vi "Quaternion to Euler.vi"(0 "Rotation Order":T2=enum."ZXY, 312", 1 "Quaternion":T3, 2 "Reference Frame":T1(ring)) -> (3 "R1":dbl, 4 "R2":dbl, 5 "R3":dbl, 6 "Singularity":bool)   [LabVIEW 2017]
uses:
  <vilib>/robotics/Kinematics/Quaternion.ctl
  <userlib>/836-Library/Sensor/IMU/Rot Order.ctl
  <vilib>/Analysis/baseanly.llb/Real Dot Product.vi
  <vilib>/Analysis/_algsub.llb/Vector Norm.vi
  <vilib>/Analysis/_algsub.llb/Real Vector Norm.vi
  <vilib>/robotics/Kinematics/Inverse Quaternion.vi
  <vilib>/robotics/Kinematics/Conjugate Quaternion.vi
  <vilib>/robotics/Kinematics/Multiply Quaternions.vi
  <vilib>/robotics/Kinematics/NI_Kinematics.lvlib
  <vilib>/Analysis/NI_AALBase.lvlib
  <vilib>/Analysis/NI_AALPro.lvlib
panel:
  out "Circular Order":bool
  out "Tait-Bryan":bool
  out "Proper Euler":bool
  # "Euler Angles"
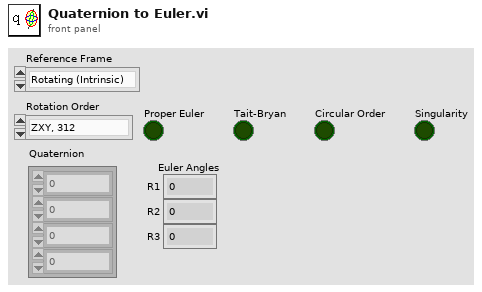
[diagram p1: front panel]
types:
  T1 = enum16{"Rotating (Intrinsic)", "Fixed (Extrinsic)"}
  T2 = typedef "Rot Order.ctl" = enum16{"ZXZ, 313", "XYX, 121", "YZY, 232", "ZYZ, 323", "XZX, 131", "YXY, 212", "XYZ, 123", "YZX, 231", "ZXY, 312", "XZY, 132", "ZYX, 321 NASA Standard Airplane", "YXZ, 213"}
  T3 = typedef "NI_Kinematics.lvlib/Quaternion.ctl" = dbl[]
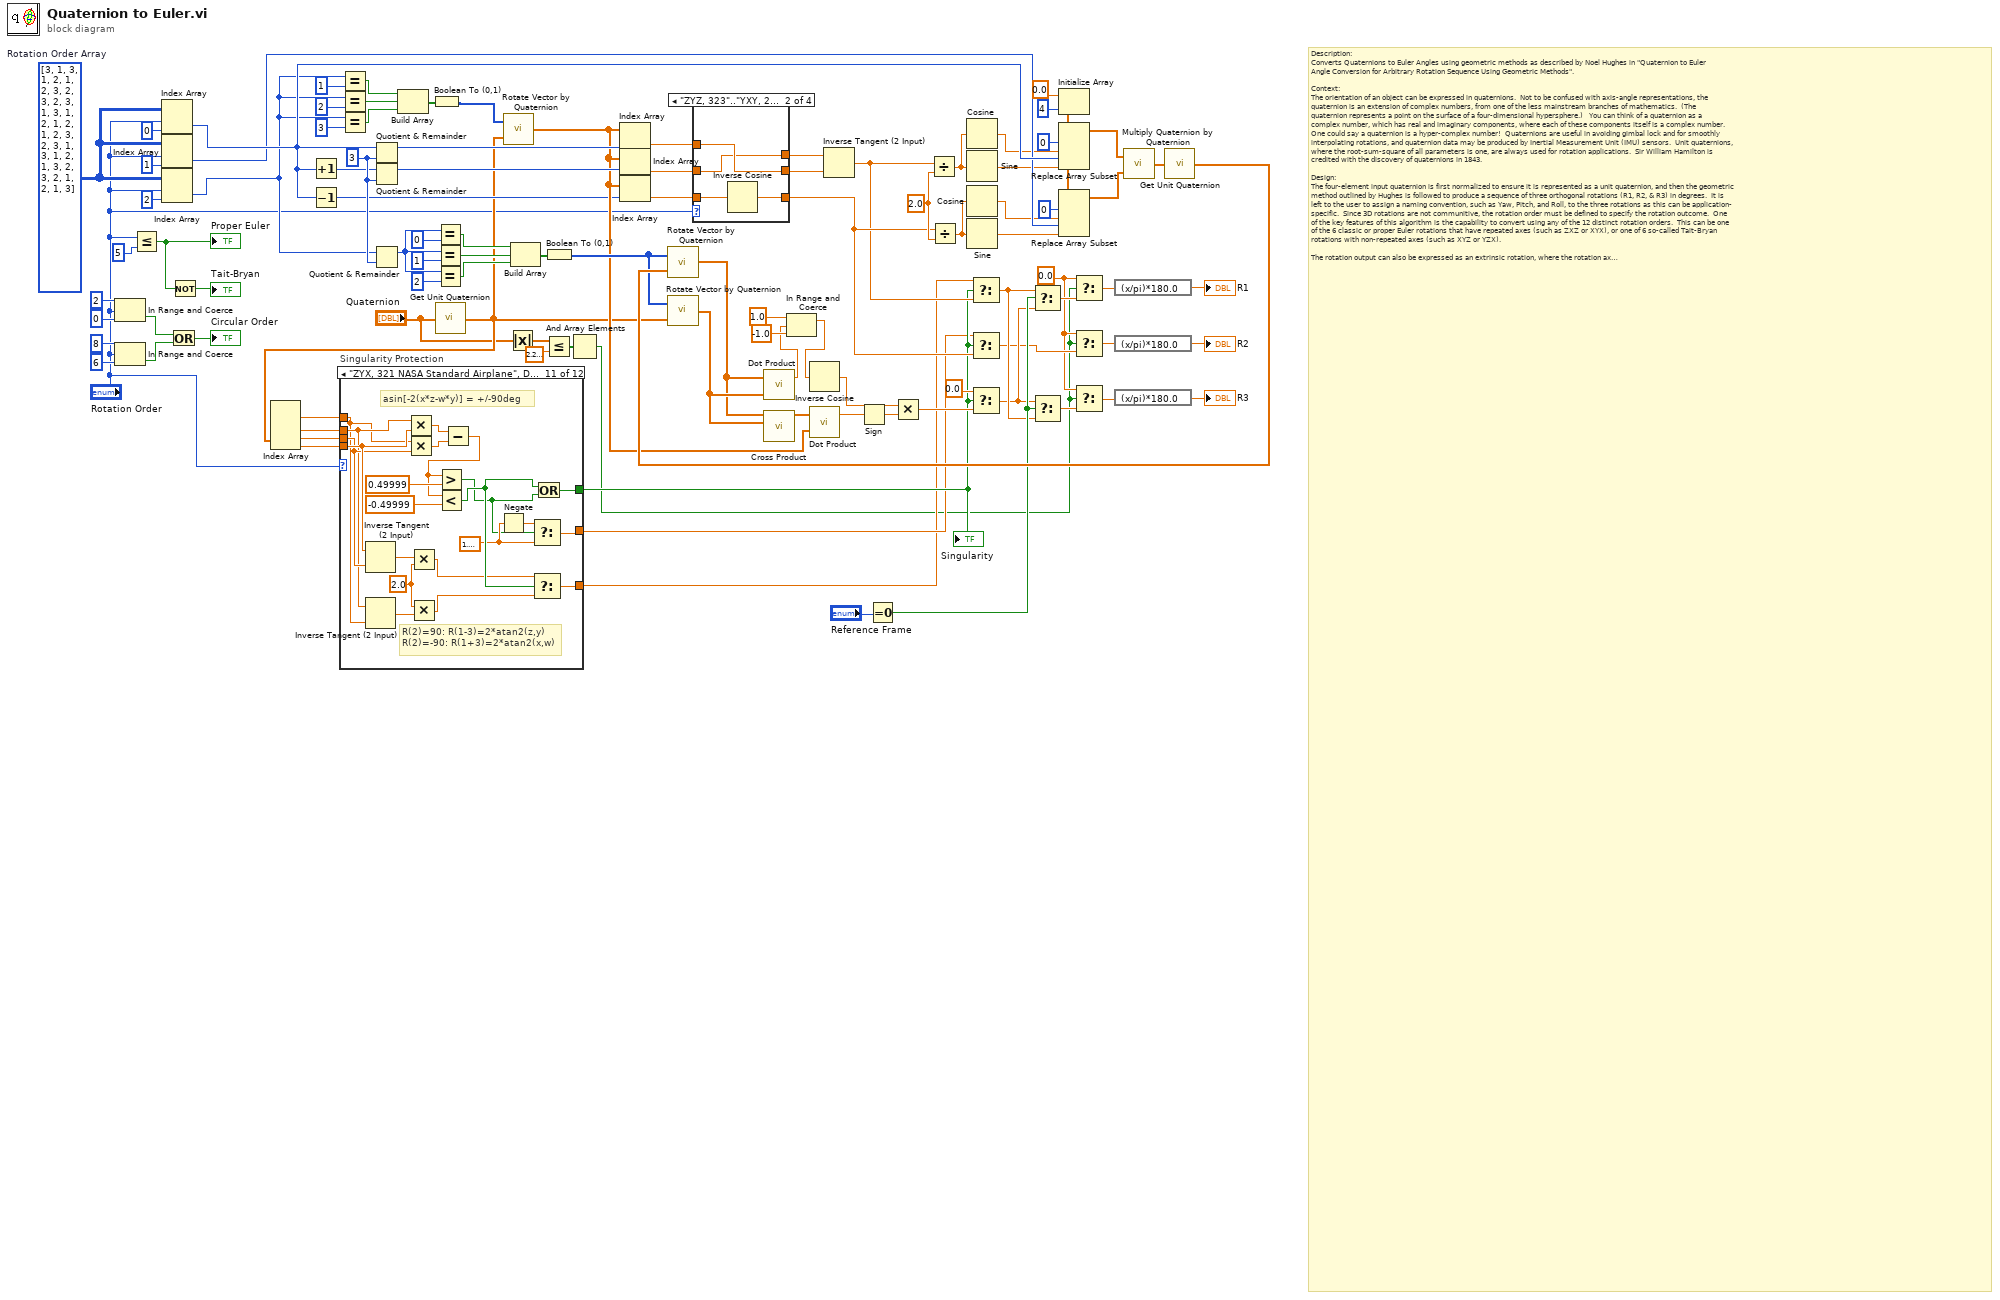
[diagram p0: block diagram]
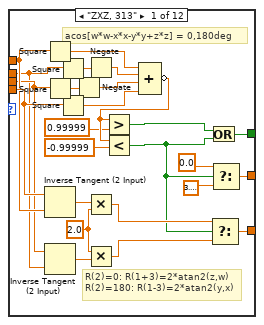
[diagram p2: hidden frame]
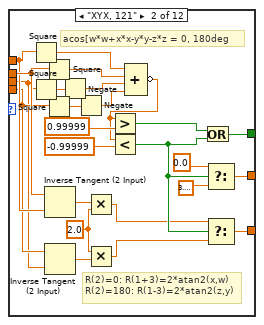
[diagram p3: hidden frame]
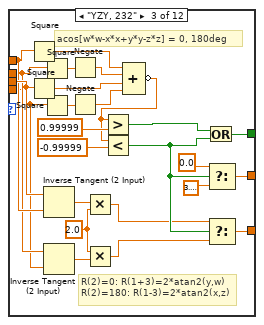
[diagram p4: hidden frame]
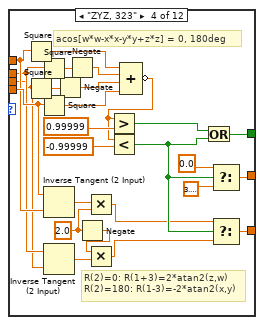
[diagram p5: hidden frame]
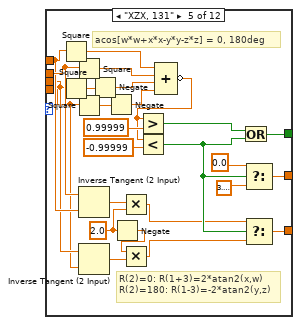
[diagram p6: hidden frame]
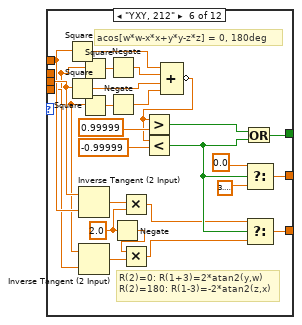
[diagram p7: hidden frame]
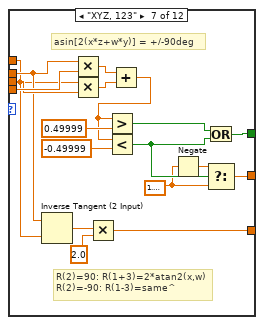
[diagram p8: hidden frame]
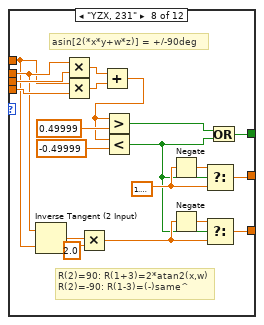
[diagram p9: hidden frame]
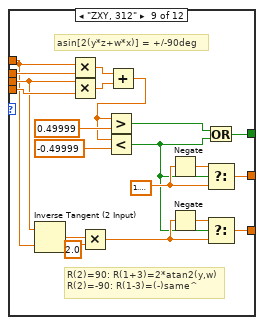
[diagram p10: hidden frame]
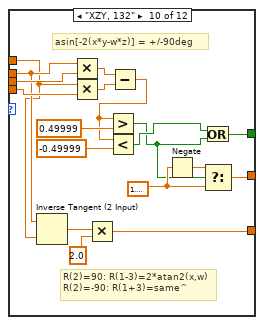
[diagram p11: hidden frame]
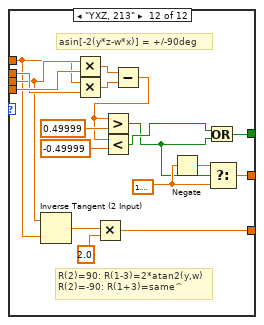
[diagram p12: hidden frame]
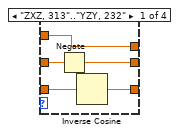
[diagram p13: hidden frame]
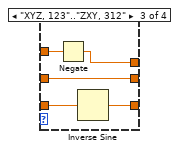
[diagram p14: hidden frame]
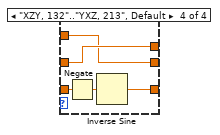
[diagram p15: hidden frame]
diagram:
  w7 = 0.0 ("t")
  w38 = 2.0 ("y")
  w75 = i16 3 ("y")
  w46 = i32[][] [[3, 1, 3], [1, 2, 1], [2, 3, 2], [3, 2, 3], [1, 3, 1], [2, 1, 2], [1, 2, 3], [2, 3, 1], [3, 1, 2], [1, 3, 2], [3, 2, 1], [2, 1, 3]]  # Rotation Order Array
  # "Description:\nConverts Quaternions to Euler Angles using geometric methods as described by Noel Hughes in \"Quaternion to Euler\nAngle Conversion for Arbitrary Rotation Sequence Using Geometric Methods\".\n\nContext:\nThe orientation of an object can be expressed in quaternions.  Not to be confused with axis-angle representations, the\nquaternion is an extension of complex numbers, from one of the less mainstream branches of mathematics.  (The\nquaternion represents a point on the surface of a four-dimensional hypersphere.)   You can think of a quaternion as a\ncomplex number, which has real and imaginary components, where each of these components itself is a complex number.\nOne could say a quaternion is a hyper-complex number!  Quaternions are useful in avoiding gimbal lock and for smoothly\ninterpolating rotations, and quaternion data may be produced by Inertial Measurement Unit (IMU) sensors.  Unit quaternions,\nwhere the root-sum-square of all parameters is one, are always used for rotation applications.  Sir William Hamilton is\ncredited with the discovery of quaternions in 1843. \n\nDesign:\nThe four-element input quaternion is first normalized to ensure it is represented as a unit quaternion, and then the geometric\nmethod outlined by Hughes is followed to produce a sequence of three orthogonal rotations (R1, R2, & R3) in degrees.  It is\nleft to the user to assign a naming convention, such as Yaw, Pitch, and Roll, to the three rotations as this can be application-\nspecific.  Since 3D rotations are not communitive, the rotation order must be defined to specify the rotation outcome.  One\nof the key features of this algorithm is the capability to convert using any of the 12 distinct rotation orders.  This can be one\nof the 6 classic or proper Euler rotations that have repeated axes (such as ZXZ or XYX), or one of 6 so-called Tait-Bryan\nrotations with non-repeated axes (such as XYZ or YZX).\n\nThe rotation output can also be expressed as an extrinsic rotation, where the rotation axes are the fixed world coordinate system,\nor an intrinsic rotation, using a coordinate system rotating with the rotating body.  Intrinsic rotations result in a changing\nreference system, where actual rotation axes might be X-Y'-Z\", for example, and are useful when the perspective is from the\nrotating body (such as an aircraft or robot).\n\nResearch determined the most elegant approach to performing this mathematically complicated conversion is described by this\nreference for a geometric conversion method by Mr. Noel Hughes:\n\n    http://www.euclideanspace.com/maths/geometry/rotations/conversions/quaternionToEuler/quat_2_euler_paper_ver2-1.pdf\n\nAll wire labels displayed in this implementation correspond to variable designations in Mr. Hughes document to facilitate\ncomparison.  Note that a different quaternion element structure is adopted here, [q0, q1i, q2j, q3k] where q0 is the real element,\nrather than [q1i, q2j, q3k, q4] where q4 is the real element (this is just a notation convention, and does not affect anything when\naccounted for).  This notation is also commonly understood as w,xi,yj,zk where 'w' is the real term coefficient.  Also note that\nequation 29 of the reference has been corrected to remove an unnecessary negative sign, and the reference equation 51 vector\nsubscript should be \"nG\" for clarity.\n\nFunctional additions to the referenced conversion approach, to provide robust coding, include :\n     (1)  a range coercion following the dot-product calculation to correct round-off error to avoid arccosine function error.\n     (2)  input value checking and mitigation for all-zero element quaternion to prevent NaN reporting in R1, R2, & R3.\n     (3)  singularity protection, which monitors for the ambiguity created when the second rotation aligns the first and third \n            rotation axes (AKA Gimbal Lock).\n\nInputs:\nQUATERNION - Input quaternion for conversion to Euler Angles.\nROTATION ORDER - Order of axis rotation used for conversion.\nREFERENCE FRAME - Designation of perspective, world coordinate system/extrinsic/fixed reference frame, or \n                                      body coordinate system/intrinsic/rotating reference frame.\n\nOutputs:\nEULER ANGLES - Cluster containing computed first, second, and third rotations (R1, R2, & R3) as converted from input quaternion. \nSINGULARITY - Boolean indicating if singularity (gimbal lock) is detected.\nPROPER EULER - Boolean indicating if rotation order is of the Proper/Classic form, (diagnostic).\nTAIT-BRYAN - Boolean indicating if rotation order is of the Tait-Bryan form, (diagnostic).\nCIRCULAR ORDER - Boolean indicating if rotation axes are in circular order, i.e. 123, 231, or 312, (diagnostic).\n\n\nVI Properties:\nExecution Reentrancy is set to Non-Reentrant Execution\n\nImplementation Considerations:\nA mathematical ambiguity can occur when the second rotation aligns the axes of the first and third rotation, also known as gimbal\nlock.  When this occurs, a degree of freedom is lost and the first and third axis rotations are indistinguishable and each produce\nthe same effect.  This is not a defect of the conversion approach or coding, but a topological result of representing 3D rotations\nwith Euler Angles.  This implementation handles the ambiguity by associating all first/third axis rotation to R1, and setting R3 to\nzero (since their respective contributions are otherwise unresolvable).  This approach is arbitrary but evidently in keeping with\ngeneral convention.  The Singularity Protection Case Structure monitors for this condition as a function of each of the 12 distinct\nrotation orders.  The way to read the notes within each case, using rotation order \"ZYX\" as an example, is:\n\n      Singularity will occur when sin[-2(x*z-w*y)] is either +90 or -90 degrees (one is Pitched North and one South).  When this\n      occurs, rotation 2 will be either +/-90 degrees, and rotations 1 and 3 are indistinguishable.  However, if R2 is +90, then we \n      know that the difference R1-R3 will equal 2*atan2(z,y).  When R2 is -90, we know that the sum R1+R3 will equal 2*atan2(x,w).\n\nEach rotation order requires a different derivation for these formulas.  The R1/R3 combination is all arbitrarily assigned to R1,\nand R3 is set to zero.  These equations were derived by this author, separately from the reference document (any errors are mine).\n\nThe implication is that under the conditions of singularity, only the second rotation R2 can be explicitly trusted to align with reality.\nThe Singularity output Boolean is available to indicate when this condition occurs.\n\n\n----- The RoboBees FRC Team 836! -----  Even hyper-complex numbers can be tamed!! ... get hyper about a career in STEM!"
  n1 = In Range and Coerce(upper limit=2, x="Rotation Order", lower limit=0) -> (In Range?=w55:bool)  [unwired: 1 out]
  n2 = In Range and Coerce(upper limit=8, x="Rotation Order", lower limit=6) -> (In Range?=w56:bool)  [unwired: 1 out]
  n3 = Less Or Equal?(x="Rotation Order", y=5) -> (x <= y?=w50:bool)
  "Proper Euler" <- w50
  n4 = Index Array(array=w46, index (row)="Rotation Order", index (col)=0 ("disabled index (col)")) -> (element=w103:i32)
  n5 = Index Array(array=w46, index (row)="Rotation Order", index (col)=1 ("disabled index (col)")) -> (element=w95:i32)
  n6 = Index Array(array=w46, index (row)="Rotation Order", index (col)=2 ("disabled index (col)")) -> (element=w74:i32)
  n7 = Or(x=w55, y=w56) -> (x .or. y?=→"Circular Order":bool)
  n8 = Not(x=w50) -> (.not. x?=→"Tait-Bryan":bool)
  n9 = Increment(x=w103) -> (x+1=w70:i32)
  n10 = Decrement(x=w103) -> (x-1=w65:i32)
  n11 = Equal?(x=w74, y=1) -> (x = y?=w62:bool)
  n12 = Equal?(x=w74, y=2) -> (x = y?=w61:bool)
  n13 = Equal?(x=w74, y=3) -> (x = y?=w63:bool)
  n14 = Quotient & Remainder(x=w103, y=w75) -> (x-y*floor(x/y)=w71:i32)  [unwired: 1 out]
  n15 = Quotient & Remainder(x=w70, y=w75) -> (x-y*floor(x/y)=w72:i32)  [unwired: 1 out]
  n16 = Quotient & Remainder(x=w74, y=w75) -> (x-y*floor(x/y)=w83:i32)  [unwired: 1 out]
  n17 = Build Array(w62, w61, w63) -> (w64:bool[])
  n18 = Boolean To (0,1)(Boolean=w64) -> (0, 1=w73:i16[])
  n19 = Equal?(x=w83, y=0) -> (x = y?=w78:bool)
  n20 = Equal?(x=w83, y=1) -> (x = y?=w79:bool)
  n21 = Equal?(x=w83, y=2) -> (x = y?=w77:bool)
  n22 = call <vilib>:"Get Unit Quaternion.vi"("quaternion"="Quaternion") -> ("unit quaternion"=w33:T3)
  n23 = Index Array(array=w33) -> (element #1=w29:dbl, element #2=w28:dbl, element #3=w30:dbl, element #4=w31:dbl)  [unwired: 4 in]
  n24 = case "Singularity Protection" shown="\"ZYX, 321 NASA Standard Airplane\", Default" "Rotation Order" {
    tunnel: w29 -> [w114 w140 w164 w192 w215 w241 w264 w283 w303 w322 w341 w361]
    tunnel: w28 -> [w112 w141 w163 w191 w216 w239 w265 w284 w311 w323 w342 w368]
    tunnel: w30 -> [w113 w138 w165 w190 w214 w242 w271 w292 w304 w330 w343 w362]
    tunnel: w31 -> [w115 w139 w162 w193 w213 w240 w272 w291 w312 w329 w344 w369]
    tunnel: [w109 w131 w155 w181 w209 w234 w259 w276 w296 w316 w335 w355] -> w21
    tunnel: [w116 w137 w166 w189 w217 w243 w261 w285 w302 w319 w345 w358] -> w20
    tunnel: [w110 w136 w161 w186 w212 w237 w263 w281 w301 w321 w340 w360] -> w22
    frame "ZXZ, 313" {
      w118 = 2.0 ("y")
      # "acos[w*w-x*x-y*y+z*z] = 0,180deg"
      # "R(2)=0: R(1+3)=2*atan2(z,w)\nR(2)=180: R(1-3)=2*atan2(y,x)"
      n25 = Square(x=w114) -> (x^2=w125:dbl)
      n26 = Square(x=w113) -> (x^2=w124:dbl)
      n27 = Inverse Tangent (2 Input)(1:w114, 2:w115) -> (0:w119:dbl)
      n28 = Inverse Tangent (2 Input)(1:w112, 2:w113) -> (0:w117:dbl)
      n29 = Square(x=w112) -> (x^2=w123:dbl)
      n30 = Square(x=w115) -> (x^2=w128:dbl)
      n31 = Negate(x=w124) -> (-x=w127:dbl)
      n32 = Negate(x=w123) -> (-x=w126:dbl)
      n33 = Multiply(x=w119, y=w118) -> (x*y=w108:dbl)
      n34 = Multiply(x=w118, y=w117) -> (x*y=w107:dbl)
      n35 = Compound Arithmetic op=ADD(w125, w126, w127, w128) -> (invert w121:dbl)
      n36 = Greater?(x=w121, y=0.99999 ("upper limit")) -> (0:w111:bool)
      n37 = Less?(x=w121, y=-0.99999 ("lower limit")) -> (x < y?=w106:bool)
      n38 = Or(x=w111, y=w106) -> (x .or. y?=w110:bool)
      n39 = Select(t=w108, s=w106, f=w107) -> (s? t:f=w116:dbl)
      n40 = Select(t=0.0 ("f"), s=w106, f=3.141592653589793) -> (s? t:f=w109:dbl)
    }
    frame "XYX, 121" {
      w143 = 2.0 ("y")
      # "R(2)=0: R(1+3)=2*atan2(x,w)\nR(2)=180: R(1-3)=2*atan2(z,y)"
      # "acos[w*w+x*x-y*y-z*z = 0, 180deg"
      n41 = Square(x=w140) -> (x^2=w152:dbl)
      n42 = Square(x=w138) -> (x^2=w151:dbl)
      n43 = Square(x=w141) -> (x^2=w148:dbl)
      n44 = Square(x=w139) -> (x^2=w150:dbl)
      n45 = Inverse Tangent (2 Input)(1:w140, 2:w141) -> (0:w144:dbl)
      n46 = Inverse Tangent (2 Input)(1:w138, 2:w139) -> (0:w142:dbl)
      n47 = Negate(x=w151) -> (-x=w153:dbl)
      n48 = Negate(x=w150) -> (-x=w149:dbl)
      n49 = Multiply(x=w144, y=w143) -> (x*y=w130:dbl)
      n50 = Multiply(x=w143, y=w142) -> (x*y=w129:dbl)
      n51 = Compound Arithmetic op=ADD(w152, w148, w153, w149) -> (invert w145:dbl)
      n52 = Greater?(x=w145, y=0.99999 ("upper limit")) -> (0:w135:bool)
      n53 = Less?(x=w145, y=-0.99999 ("lower limit")) -> (x < y?=w133:bool)
      n54 = Or(x=w135, y=w133) -> (x .or. y?=w136:bool)
      n55 = Select(t=0.0 ("f"), s=w133, f=3.141592653589793) -> (s? t:f=w131:dbl)
      n56 = Select(t=w130, s=w133, f=w129) -> (s? t:f=w137:dbl)
    }
    frame "YZY, 232" {
      w168 = 2.0 ("y")
      # "R(2)=0: R(1+3)=2*atan2(y,w)\nR(2)=180: R(1-3)=2*atan2(x,z)"
      # "acos[w*w-x*x+y*y-z*z] = 0, 180deg"
      n57 = Square(x=w164) -> (x^2=w177:dbl)
      n58 = Square(x=w165) -> (x^2=w173:dbl)
      n59 = Square(x=w163) -> (x^2=w176:dbl)
      n60 = Square(x=w162) -> (x^2=w175:dbl)
      n61 = Inverse Tangent (2 Input)(1:w164, 2:w165) -> (0:w169:dbl)
      n62 = Inverse Tangent (2 Input)(1:w162, 2:w163) -> (0:w167:dbl)
      n63 = Negate(x=w176) -> (-x=w178:dbl)
      n64 = Negate(x=w175) -> (-x=w174:dbl)
      n65 = Multiply(x=w169, y=w168) -> (x*y=w157:dbl)
      n66 = Multiply(x=w168, y=w167) -> (x*y=w156:dbl)
      n67 = Compound Arithmetic op=ADD(w177, w178, w173, w174) -> (invert w170:dbl)
      n68 = Greater?(x=w170, y=0.99999 ("upper limit")) -> (0:w160:bool)
      n69 = Less?(x=w170, y=-0.99999 ("lower limit")) -> (x < y?=w158:bool)
      n70 = Or(x=w160, y=w158) -> (x .or. y?=w161:bool)
      n71 = Select(t=0.0 ("f"), s=w158, f=3.141592653589793) -> (s? t:f=w155:dbl)
      n72 = Select(t=w157, s=w158, f=w156) -> (s? t:f=w166:dbl)
    }
    frame "ZYZ, 323" {
      w188 = 2.0 ("y")
      # "R(2)=0: R(1+3)=2*atan2(z,w)\nR(2)=180: R(1-3)=-2*atan2(x,y)"
      # "acos[w*w-x*x-y*y+z*z] = 0, 180deg"
      n73 = Square(x=w192) -> (x^2=w201:dbl)
      n74 = Square(x=w190) -> (x^2=w200:dbl)
      n75 = Square(x=w191) -> (x^2=w199:dbl)
      n76 = Square(x=w193) -> (x^2=w204:dbl)
      n77 = Inverse Tangent (2 Input)(1:w192, 2:w193) -> (0:w195:dbl)
      n78 = Inverse Tangent (2 Input)(1:w190, 2:w191) -> (0:w194:dbl)
      n79 = Negate(x=w200) -> (-x=w203:dbl)
      n80 = Negate(x=w199) -> (-x=w202:dbl)
      n81 = Negate(x=w188) -> (-x=w187:dbl)
      n82 = Multiply(x=w195, y=w188) -> (x*y=w180:dbl)
      n83 = Multiply(x=w187, y=w194) -> (x*y=w179:dbl)
      n84 = Compound Arithmetic op=ADD(w201, w202, w203, w204) -> (invert w196:dbl)
      n85 = Greater?(x=w196, y=0.99999 ("upper limit")) -> (0:w185:bool)
      n86 = Less?(x=w196, y=-0.99999 ("lower limit")) -> (x < y?=w183:bool)
      n87 = Or(x=w185, y=w183) -> (x .or. y?=w186:bool)
      n88 = Select(t=0.0 ("f"), s=w183, f=3.141592653589793) -> (s? t:f=w181:dbl)
      n89 = Select(t=w180, s=w183, f=w179) -> (s? t:f=w189:dbl)
    }
    frame "XZX, 131" {
      w219 = 2.0 ("y")
      # "R(2)=0: R(1+3)=2*atan2(x,w)\nR(2)=180: R(1-3)=-2*atan2(y,z)"
      # "acos[w*w+x*x-y*y-z*z] = 0, 180deg"
      n90 = Square(x=w215) -> (x^2=w229:dbl)
      n91 = Square(x=w214) -> (x^2=w228:dbl)
      n92 = Square(x=w216) -> (x^2=w225:dbl)
      n93 = Square(x=w213) -> (x^2=w227:dbl)
      n94 = Inverse Tangent (2 Input)(1:w215, 2:w216) -> (0:w221:dbl)
      n95 = Inverse Tangent (2 Input)(1:w213, 2:w214) -> (0:w220:dbl)
      n96 = Negate(x=w228) -> (-x=w230:dbl)
      n97 = Negate(x=w227) -> (-x=w226:dbl)
      n98 = Negate(x=w219) -> (-x=w218:dbl)
      n99 = Multiply(x=w221, y=w219) -> (x*y=w206:dbl)
      n100 = Multiply(x=w218, y=w220) -> (x*y=w205:dbl)
      n101 = Compound Arithmetic op=ADD(w229, w225, w230, w226) -> (invert w222:dbl)
      n102 = Greater?(x=w222, y=0.99999 ("upper limit")) -> (0:w211:bool)
      n103 = Less?(x=w222, y=-0.99999 ("lower limit")) -> (x < y?=w208:bool)
      n104 = Or(x=w211, y=w208) -> (x .or. y?=w212:bool)
      n105 = Select(t=0.0 ("f"), s=w208, f=3.141592653589793) -> (s? t:f=w209:dbl)
      n106 = Select(t=w206, s=w208, f=w205) -> (s? t:f=w217:dbl)
    }
    frame "YXY, 212" {
      w245 = 2.0 ("y")
      # "R(2)=0: R(1+3)=2*atan2(y,w)\nR(2)=180: R(1-3)=-2*atan2(z,x)"
      # "acos[w*w-x*x+y*y-z*z] = 0, 180deg"
      n107 = Square(x=w241) -> (x^2=w255:dbl)
      n108 = Square(x=w242) -> (x^2=w251:dbl)
      n109 = Inverse Tangent (2 Input)(1:w241, 2:w242) -> (0:w247:dbl)
      n110 = Inverse Tangent (2 Input)(1:w239, 2:w240) -> (0:w246:dbl)
      n111 = Square(x=w239) -> (x^2=w254:dbl)
      n112 = Square(x=w240) -> (x^2=w253:dbl)
      n113 = Negate(x=w254) -> (-x=w256:dbl)
      n114 = Negate(x=w253) -> (-x=w252:dbl)
      n115 = Negate(x=w245) -> (-x=w244:dbl)
      n116 = Multiply(x=w247, y=w245) -> (x*y=w232:dbl)
      n117 = Multiply(x=w244, y=w246) -> (x*y=w231:dbl)
      n118 = Compound Arithmetic op=ADD(w255, w256, w251, w252) -> (invert w248:dbl)
      n119 = Greater?(x=w248, y=0.99999 ("upper limit")) -> (0:w238:bool)
      n120 = Less?(x=w248, y=-0.99999 ("lower limit")) -> (x < y?=w233:bool)
      n121 = Or(x=w238, y=w233) -> (x .or. y?=w237:bool)
      n122 = Select(t=0.0 ("f"), s=w233, f=3.141592653589793) -> (s? t:f=w234:dbl)
      n123 = Select(t=w232, s=w233, f=w231) -> (s? t:f=w243:dbl)
    }
    frame "XYZ, 123" {
      w257 = 1.5707963267948966
      # "R(2)=90: R(1+3)=2*atan2(x,w)\nR(2)=-90: R(1-3)=same^"
      # "asin[2(x*z+w*y)] = +/-90deg"
      n124 = Inverse Tangent (2 Input)(1:w264, 2:w265) -> (0:w267:dbl)
      n125 = Multiply(x=w265, y=w272) -> (x*y=w274:dbl)
      n126 = Multiply(x=w264, y=w271) -> (x*y=w273:dbl)
      n127 = Multiply(x=w267, y=2.0) -> (x*y=w261:dbl)
      n128 = Add(x=w274, y=w273) -> (x+y=w268:dbl)
      n129 = Greater?(x=w268, y=0.49999 ("upper limit")) -> (0:w262:bool)
      n130 = Less?(x=w268, y=-0.49999 ("lower limit")) -> (x < y?=w260:bool)
      n131 = Negate(x=w257) -> (-x=w258:dbl)
      n132 = Or(x=w262, y=w260) -> (x .or. y?=w263:bool)
      n133 = Select(t=w258, s=w260, f=w257) -> (s? t:f=w259:dbl)
    }
    frame "YZX, 231" {
      w277 = 1.5707963267948966
      # "R(2)=90: R(1+3)=2*atan2(x,w)\nR(2)=-90: R(1-3)=(-)same^"
      # "asin[2(*x*y+w*z)] = +/-90deg"
      n134 = Inverse Tangent (2 Input)(1:w283, 2:w284) -> (0:w287:dbl)
      n135 = Multiply(x=w284, y=w292) -> (x*y=w293:dbl)
      n136 = Multiply(x=w283, y=w291) -> (x*y=w294:dbl)
      n137 = Multiply(x=w287, y=2.0) -> (x*y=w279:dbl)
      n138 = Add(x=w293, y=w294) -> (x+y=w288:dbl)
      n139 = Greater?(x=w288, y=0.49999 ("upper limit")) -> (0:w280:bool)
      n140 = Less?(x=w288, y=-0.49999 ("lower limit")) -> (x < y?=w275:bool)
      n141 = Negate(x=w277) -> (-x=w278:dbl)
      n142 = Negate(x=w279) -> (-x=w282:dbl)
      n143 = Select(t=w278, s=w275, f=w277) -> (s? t:f=w276:dbl)
      n144 = Select(t=w282, s=w275, f=w279) -> (s? t:f=w285:dbl)
      n145 = Or(x=w280, y=w275) -> (x .or. y?=w281:bool)
    }
    frame "ZXY, 312" {
      w297 = 1.5707963267948966
      # "R(2)=90: R(1+3)=2*atan2(y,w)\nR(2)=-90: R(1-3)=(-)same^"
      # "asin[2(y*z+w*x)] = +/-90deg"
      n146 = Inverse Tangent (2 Input)(1:w303, 2:w304) -> (0:w307:dbl)
      n147 = Multiply(x=w303, y=w311) -> (x*y=w314:dbl)
      n148 = Multiply(x=w304, y=w312) -> (x*y=w313:dbl)
      n149 = Multiply(x=w307, y=2.0) -> (x*y=w299:dbl)
      n150 = Add(x=w314, y=w313) -> (x+y=w308:dbl)
      n151 = Greater?(x=w308, y=0.49999 ("upper limit")) -> (0:w300:bool)
      n152 = Less?(x=w308, y=-0.49999 ("lower limit")) -> (x < y?=w295:bool)
      n153 = Negate(x=w297) -> (-x=w298:dbl)
      n154 = Negate(x=w299) -> (-x=w305:dbl)
      n155 = Or(x=w300, y=w295) -> (x .or. y?=w301:bool)
      n156 = Select(t=w298, s=w295, f=w297) -> (s? t:f=w296:dbl)
      n157 = Select(t=w305, s=w295, f=w299) -> (s? t:f=w302:dbl)
    }
    frame "XZY, 132" {
      w317 = 1.5707963267948966
      # "R(2)=90: R(1-3)=2*atan2(x,w)\nR(2)=-90: R(1+3)=same^"
      # "asin[-2(x*y-w*z)] = +/-90deg"
      n158 = Inverse Tangent (2 Input)(1:w322, 2:w323) -> (0:w325:dbl)
      n159 = Multiply(x=w323, y=w330) -> (x*y=w332:dbl)
      n160 = Multiply(x=w322, y=w329) -> (x*y=w331:dbl)
      n161 = Multiply(x=w325, y=2.0) -> (x*y=w319:dbl)
      n162 = Subtract(x=w332, y=w331) -> (x-y=w326:dbl)
      n163 = Greater?(x=w326, y=0.49999 ("upper limit")) -> (0:w315:bool)
      n164 = Less?(x=w326, y=-0.49999 ("lower limit")) -> (x < y?=w320:bool)
      n165 = Negate(x=w317) -> (-x=w318:dbl)
      n166 = Or(x=w320, y=w315) -> (x .or. y?=w321:bool)
      n167 = Select(t=w318, s=w315, f=w317) -> (s? t:f=w316:dbl)
    }
    frame "ZYX, 321 NASA Standard Airplane", Default {
      w337 = 1.5707963267948966
      w347 = 2.0 ("y")
      # "R(2)=90: R(1-3)=2*atan2(z,y)\nR(2)=-90: R(1+3)=2*atan2(x,w)"
      # "asin[-2(x*z-w*y)] = +/-90deg"
      n168 = Inverse Tangent (2 Input)(1:w343, 2:w344) -> (0:w348:dbl)
      n169 = Inverse Tangent (2 Input)(1:w341, 2:w342) -> (0:w346:dbl)
      n170 = Multiply(x=w342, y=w344) -> (x*y=w352:dbl)
      n171 = Multiply(x=w341, y=w343) -> (x*y=w353:dbl)
      n172 = Multiply(x=w348, y=w347) -> (x*y=w334:dbl)
      n173 = Multiply(x=w347, y=w346) -> (x*y=w333:dbl)
      n174 = Subtract(x=w352, y=w353) -> (x-y=w349:dbl)
      n175 = Greater?(x=w349, y=0.49999 ("upper limit")) -> (0:w336:bool)
      n176 = Less?(x=w349, y=-0.49999 ("lower limit")) -> (x < y?=w339:bool)
      n177 = Negate(x=w337) -> (-x=w338:dbl)
      n178 = Select(t=w338, s=w336, f=w337) -> (s? t:f=w335:dbl)
      n179 = Select(t=w334, s=w339, f=w333) -> (s? t:f=w345:dbl)
      n180 = Or(x=w339, y=w336) -> (x .or. y?=w340:bool)
    }
    frame "YXZ, 213" {
      w356 = 1.5707963267948966
      # "R(2)=90: R(1-3)=2*atan2(y,w)\nR(2)=-90: R(1+3)=same^"
      # "asin[-2(y*z-w*x)] = +/-90deg"
      n181 = Inverse Tangent (2 Input)(1:w361, 2:w362) -> (0:w364:dbl)
      n182 = Multiply(x=w362, y=w369) -> (x*y=w370:dbl)
      n183 = Multiply(x=w361, y=w368) -> (x*y=w371:dbl)
      n184 = Multiply(x=w364, y=2.0) -> (x*y=w358:dbl)
      n185 = Subtract(x=w370, y=w371) -> (x-y=w365:dbl)
      n186 = Greater?(x=w365, y=0.49999 ("upper limit")) -> (0:w354:bool)
      n187 = Less?(x=w365, y=-0.49999 ("lower limit")) -> (x < y?=w359:bool)
      n188 = Negate(x=w356) -> (-x=w357:dbl)
      n189 = Or(x=w359, y=w354) -> (x .or. y?=w360:bool)
      n190 = Select(t=w357, s=w354, f=w356) -> (s? t:f=w355:dbl)
    }
  }
  "Singularity" <- w22
  n191 = call <vilib>:"Rotate Vector by Quaternion.vi"("quaternion"=w33, "vector"=w73) -> ("rotated vector"=w67:dbl[])  [unwired: 1 in]
  n192 = Absolute Value(x="Quaternion") -> (abs(x)=w1:T3)
  n193 = Build Array(w78, w79, w77) -> (w76:bool[])
  n194 = Boolean To (0,1)(Boolean=w76) -> (0, 1=w84:i16[])
  n195 = Less Or Equal?(x=w1, y=2.220446049250313e-16) -> (x <= y?=w14:bool[])
  n196 = And Array Elements(Boolean array=w14) -> (logical AND=w3:bool)
  n197 = Index Array(array=w67, index=w71) -> (element=w68:dbl)
  n198 = Index Array(array=w67, index=w72) -> (element=w101:dbl)
  n199 = Index Array(array=w67, index=w65) -> (element=w66:dbl)
  n200 = call <vilib>:"Rotate Vector by Quaternion.vi"("quaternion"=w33, "vector"=w84) -> ("rotated vector"=w40:dbl[])  [unwired: 1 in]
  n201 = case shown="\"ZYZ, 323\"..\"YXY, 212\"" "Rotation Order" {
    tunnel: w66 -> [w374 w380 w381 w389]
    tunnel: w68 -> [w373 w378 w385 w386]
    tunnel: [w373 w377 w384 w387] -> w69
    tunnel: [w372 w379 w382 w390] -> w24
    tunnel: w101 -> [w376 w377 w383 w387]
    tunnel: [w375 w378 w383 w386] -> w102
    frame "ZXZ, 313".."YZY, 232" {
      n202 = Negate(x=w376) -> (-x=w375:dbl)
      n203 = Inverse Cosine(1:w374) -> (0:w372:dbl)
    }
    frame "ZYZ, 323".."YXY, 212" {
      n204 = Inverse Cosine(1:w380) -> (0:w379:dbl)
    }
    frame "XYZ, 123".."ZXY, 312" {
      n205 = Negate(x=w385) -> (-x=w384:dbl)
      n206 = Inverse Sine(1:w381) -> (0:w382:dbl)
    }
    frame "XZY, 132".."YXZ, 213", Default {
      n207 = Negate(x=w389) -> (-x=w388:dbl)
      n208 = Inverse Sine(1:w388) -> (0:w390:dbl)
    }
  }
  n209 = Inverse Tangent (2 Input)(1:w102, 2:w69) -> (0:w23:dbl)
  n210 = Equal To 0?(x="Reference Frame") -> (x = 0?=w18:bool)
  n211 = Divide(x=w23, y=w38) -> (x/y=w87:dbl)
  n212 = Divide(x=w24, y=w38) -> (x/y=w92:dbl)
  n213 = Cosine(x=w87) -> (cos(x)=w86:dbl)
  n214 = Sine(x=w87) -> (sin(x)=w85:dbl)
  n215 = Cosine(x=w92) -> (cos(x)=w93:dbl)
  n216 = Sine(x=w92) -> (sin(x)=w94:dbl)
  n217 = Select(t=w20, s=w22, f=w23) -> (s? t:f=w17:dbl)
  n218 = Select(t=w21, s=w22, f=w24) -> (s? t:f=w9:dbl)
  n219 = Initialize Array(0.0 ("element"), 4 ("dimension size")) -> (w96:dbl[])
  n220 = Replace Array Subset(array=w96, new element #1=w86, index #1=0 ("index"), new element #2=w85, index #2=w103) -> (w97:dbl[])
  n221 = Replace Array Subset(array=w96, new element #1=w93, index #1=0 ("index"), new element #2=w94, index #2=w95) -> (w98:dbl[])
  n222 = Select(t=w7, s=w3, f=w9) -> (s? t:f=w5:dbl)
  n223 = expression code="(x/pi)*180.0" ("rads to degs")(w5) -> (→"R2":dbl)
  n224 = call <vilib>:"Multiply Quaternion by Quaternion.vi"("y"=w98, "quaternion"=w97) -> ("product"=w99:T3)
  n225 = call <vilib>:"Get Unit Quaternion.vi"("quaternion"=w99) -> ("unit quaternion"=w100:T3)
  n226 = call <vilib>:"Rotate Vector by Quaternion.vi"("quaternion"=w100, "vector"=w84) -> ("rotated vector"=w39:dbl[])  [unwired: 1 in]
  n227 = call-poly <vilib>:"Dot Product.vi"("Y Vector"=w40, "X Vector"=w39) -> ("X * Y"=w35:dbl)  [unwired: 1 out]
  n228 = call <vilib>:"Cross Product.vi"("B Vector"=w40, "A Vector"=w39) -> ("Cross Product"=w41:dbl[])  [unwired: 8 in, 1 out]
  n229 = In Range and Coerce(upper limit=1.0, x=w35, lower limit=-1.0 ("y")) -> (coerced(x)=w34:dbl)  [unwired: 1 out]
  n230 = Inverse Cosine(1:w34) -> (0:w27:dbl)
  n231 = call-poly <vilib>:"Dot Product.vi"("Y Vector"=w67, "X Vector"=w41) -> ("X * Y"=w42:dbl)  [unwired: 1 out]
  n232 = Sign(1:w42) -> (0:w43:dbl)
  n233 = Multiply(x=w27, y=w43) -> (x*y=w25:dbl)
  n234 = Select(t=0.0, s=w22, f=w25) -> (s? t:f=w16:dbl)
  n235 = Select(t=w17, s=w18, f=w16) -> (s? t:f=w10:dbl)
  n236 = Select(t=w16, s=w18, f=w17) -> (s? t:f=w8:dbl)
  n237 = Select(t=w7, s=w3, f=w10) -> (s? t:f=w6:dbl)
  n238 = Select(t=w7, s=w3, f=w8) -> (s? t:f=w4:dbl)
  n239 = expression code="(x/pi)*180.0" ("rads to degs")(w6) -> (→"R1":dbl)
  n240 = expression code="(x/pi)*180.0" ("rads to degs")(w4) -> (→"R3":dbl)
